vi "Get Device Config.vi"(1 "Device ID":u8, 2 "Device Family":T2) -> (0 "Channels":T1)   [LabVIEW 2011, in "LVH-LINX.lvlib"]
uses:
  LVH-LINX.lvlib
  Type Defs/Device Family.ctl
  Type Defs/Devices/Generic Device.ctl
  Type Defs/Devices - NI.ctl
  Type Defs/Devices - Digilent.ctl
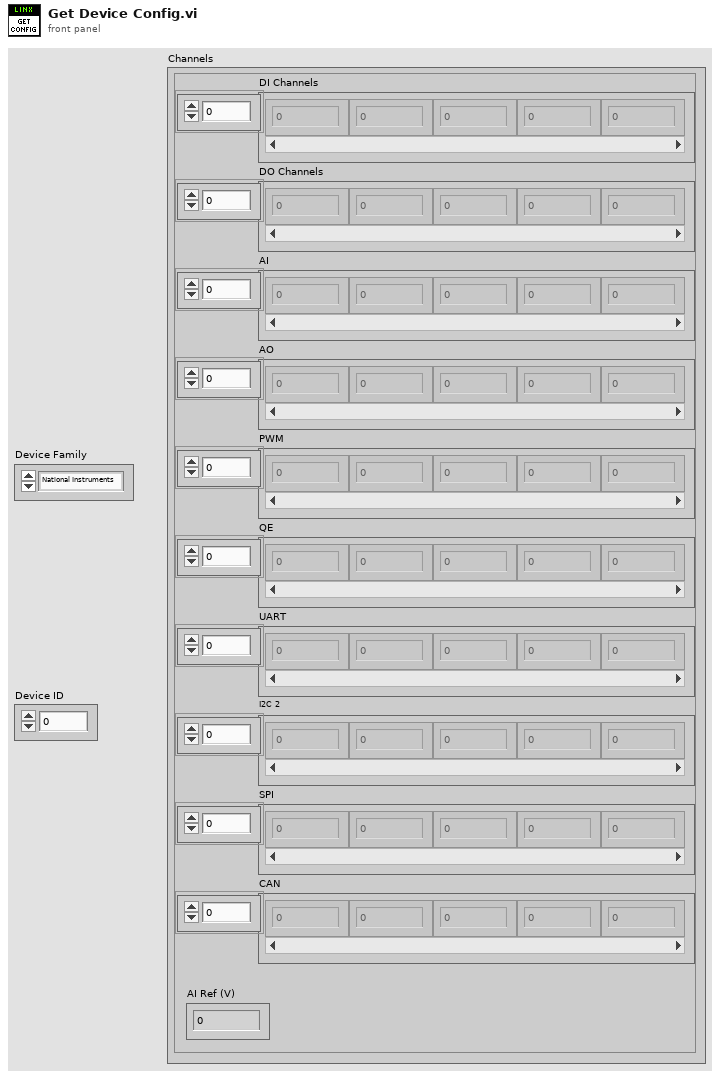
[diagram p1: front panel]
types:
  T1 = typedef "LVH-LINX.lvlib/Generic Device.ctl" = cluster{"DI Channels":u8[], "DO Channels":u8[], "AI":u8[], "AO":u8[], "PWM":u8[], "QE":u8[], "UART":u8[], "I2C 2":u8[], "SPI":u8[], "CAN":u8[], "AI Ref (V)":dbl}
  T2 = typedef "LVH-LINX.lvlib/Device Family.ctl" = enum8{"National Instruments", "Digilent", "Arduino"}
  T3 = typedef "LVH-LINX.lvlib/Devices - NI.ctl" = enum16{"myRIO-1900", "myRIO-1950"}
  T4 = typedef "LVH-LINX.lvlib/Devices - Digilent.ctl" = enum16{"chipKIT Uno32", "chipKIT uC32", "chipKIT Max32", "chipKIT DP32"}
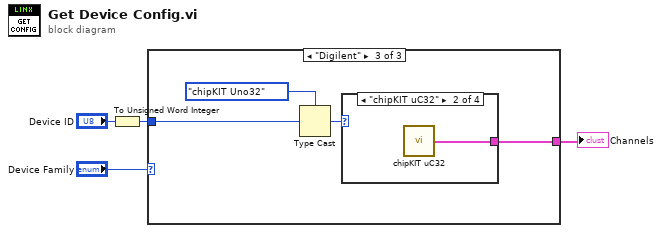
[diagram p0: block diagram]
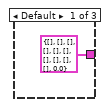
[diagram p2: hidden frame]
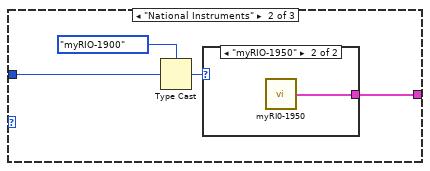
[diagram p3: hidden frame]
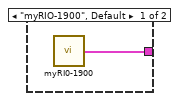
[diagram p4: hidden frame]
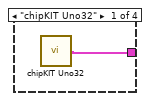
[diagram p5: hidden frame]
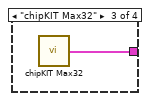
[diagram p6: hidden frame]
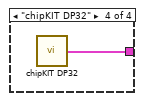
[diagram p7: hidden frame]
diagram:
  n1 = To Unsigned Word Integer(number="Device ID") -> (unsigned 16bit integer=w1:u16)
  n2 = case shown="\"Digilent\"" "Device Family" {
    tunnel: [T1 {"DI Channels"=[], "DO Channels"=[], "AI"=[], "AO"=[], "PWM"=[], "QE"=[], "UART"=[], "I2C 2"=[], "SPI"=[], "CAN"=[], "AI Ref (V)"=0.0} ("chipKIT DP32") w7 w14] -> w3
    tunnel: w1 -> [_ w6 w12]
    frame Default {
    }
    frame "National Instruments" {
      n3 = Type Cast(type=Devices_-_NI."myRIO-1900" ("NI Device"), x=w6) -> (*(type *) &x=w8:T3)
      n4 = case shown="\"myRIO-1950\"" w8 {
        tunnel: [w10 w11] -> w7
        frame "myRIO-1900", Default {
          n5 = call "myRI0-1900.vi"() -> ("myRIO-1900"=w10:T1)
        }
        frame "myRIO-1950" {
          n6 = call "myRI0-1950.vi"() -> ("myRIO-1900"=w11:T1)
        }
      }
    }
    frame "Digilent" {
      n7 = Type Cast(type=Devices_-_Digilent."chipKIT Uno32" ("Digilent Device"), x=w12) -> (*(type *) &x=w15:T4)
      n8 = case shown="\"chipKIT uC32\"" w15 {
        tunnel: [w16 w17 w18 w19] -> w14
        frame "chipKIT Uno32" {
          n9 = call "chipKIT Uno32.vi"() -> ("chipKIT Uno32"=w16:T1)
        }
        frame "chipKIT uC32" {
          n10 = call "chipKIT uC32.vi"() -> ("chipKIT uC32"=w17:T1)
        }
        frame "chipKIT Max32" {
          n11 = call "chipKIT Max32.vi"() -> ("chipKIT Max32"=w18:T1)
        }
        frame "chipKIT DP32" {
          n12 = call "chipKIT DP32.vi"() -> ("chipKIT DP32"=w19:T1)
        }
      }
    }
  }
  "Channels" <- w3
